vi "Test Convert Current Time to RFC3339Nano.vi"(8 "error in (no error)":errorcluster) -> (0 "error out":errorcluster)   [LabVIEW 2017, in "UT_LokiJsonFormatter.lvlib"]
doc: "Template for an unit test with caraya in the \"Given, When, Then\" structure from James."
uses:
  UT_LokiJsonFormatter.lvlib
  <vilib>/addons/_JKI Toolkits/Caraya/classes/Assert/Assert Greater_Variant.vi
  <vilib>/addons/_JKI Toolkits/Caraya/classes/Test/Test.lvclass
  <vilib>/addons/_JKI Toolkits/Caraya/classes/Assert/Assert.lvclass
  Source/HSE-Logger/Formatter/LokiJsonFormatter/LokiJsonFormatter.lvclass
panel:
  # "Connector Pane"
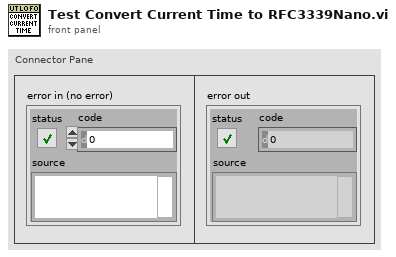
[diagram p1: front panel]
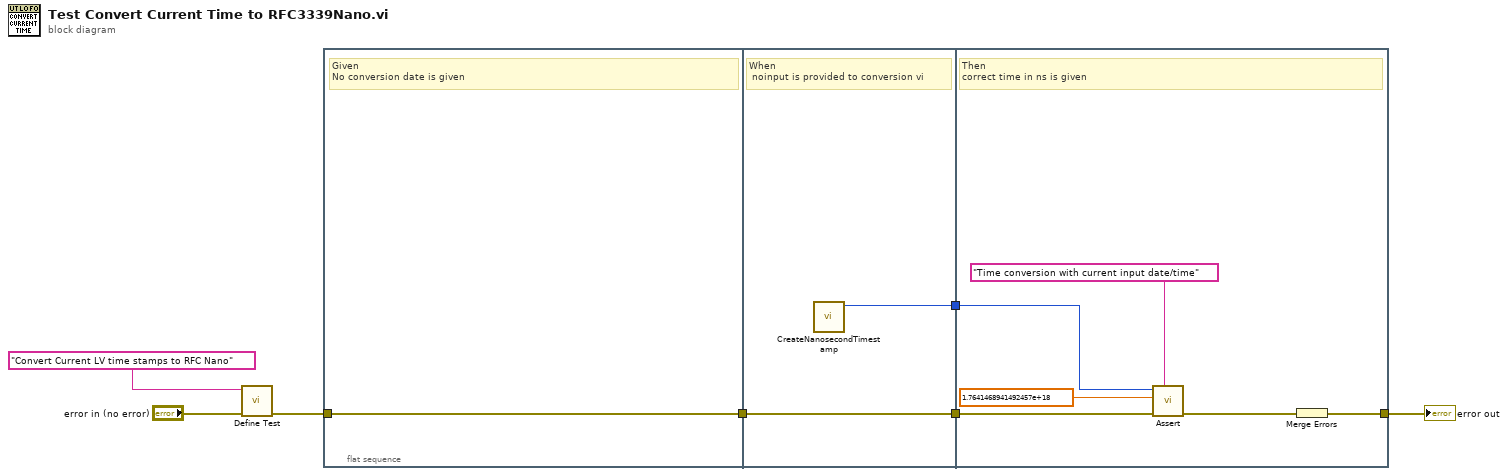
[diagram p0: block diagram]
diagram:
  n1 = call <vilib>:"Define Test.vi"("error in (no error)"="error in (no error)", "Label (VI Title)"="Convert Current LV time stamps to RFC Nano") -> ("error out"=w4:errorcluster)  [unwired: 8 in, 1 out]
  n2 = flat-sequence {
    tunnel: w4 -> [w8]
    tunnel: [w8] -> w7
    tunnel: w7 -> [w10]
    tunnel: [w10] -> w2
    tunnel: [w9] -> w1
    tunnel: [w15] -> w6
    tunnel: w2 -> [w14]
    tunnel: w1 -> [w11]
    frame #0 {
      # "Given\nNo conversion date is given"
    }
    frame #1 {
      # "When\n noinput is provided to conversion vi"
      n3 = call "CreateNanosecondTimestamp.vi"() -> ("Time in RFC3339Nano"=w9:i64)  [unwired: 10 in, 1 out]
    }
    frame #2 {
      # "Then\ncorrect time in ns is given"
      n4 = call-poly <vilib>:"Assert.vi"("Label"="Time conversion with current input date/time", "error in (no error)"=w14, "Actual"=1.7641468941492457e+18, "Expected"=w11) -> ("error out"=w16:errorcluster)  [unwired: 6 in, 1 out]
      n5 = Merge Errors(w16) -> (w15:errorcluster)
    }
  }
  "error out" <- w6
